vi "FindBlob_Pass1.vi"(0 "Image in":u32[][](graph), 1 "Connectivity":enum16{"4", "8"}(ring)) -> (2 "Image out":u32[][](graph), 3 "output array":u32[](array[numeric]), 4 "duplicates":cluster{u8, u8, u8}[](array[cluster]))   [LabVIEW 2024]
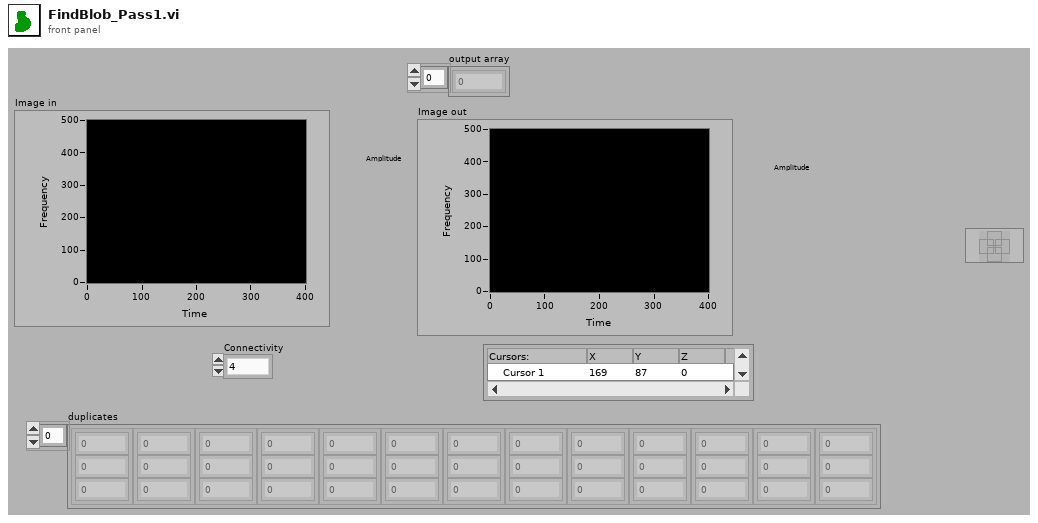
[diagram p1: front panel]
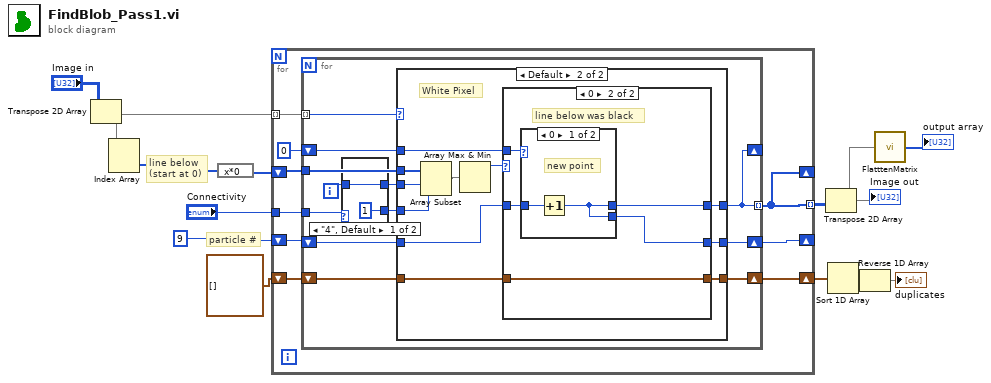
[diagram p0: block diagram]
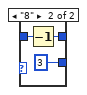
[diagram p2: hidden frame]
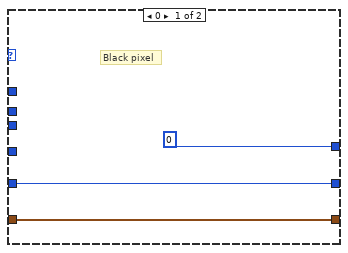
[diagram p3: hidden frame]
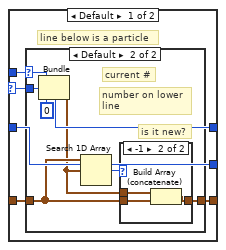
[diagram p4: hidden frame]
diagram:
  # "particle #"
  # "line below\n(start at 0)"
  n1 = Transpose 2D Array(2D array="Image in") -> (transposed array=w8:u32[][])
  n2 = Index Array(array=w8) -> (element=w9:u32[])  [unwired: 2 in]
  n3 = expression code="x*0"(w9) -> (w10:u32[])
  n4 = for {
    tunnel: w8 -> [w20] mode=indexing
    shift-right: [w21] -> _
    shift-left: u32 9 -> [w22]
    tunnel: [w18] -> w6 mode=indexing
    shift-right: [w18] -> _
    shift-left: w10 -> [w19]
    tunnel: "Connectivity" -> [w17]
    shift-right: [w15] -> w13
    shift-left: cluster{u8, u8, u8}[] [] -> [w16]
    n5 = for {
      tunnel: w20 -> [w34] mode=indexing
      shift-right: [w23] -> _
      shift-left: u32 0 -> [w33]
      shift-right: [w32] -> w21
      shift-left: w22 -> [w31]
      tunnel: [w23] -> w18 mode=indexing
      tunnel: w19 -> [w30]
      tunnel: w17 -> [w26]
      shift-right: [w24] -> w15
      shift-left: w16 -> [w25]
      i -> [w29]
      n6 = case shown="\"4\", Default" w26 {
        tunnel: w29 -> [w36 w39]
        tunnel: [w36 w38] -> w28
        tunnel: [1 ("length") 3 ("length")] -> w27
        frame "4", Default {
        }
        frame "8" {
          n7 = Decrement(x=w39) -> (x-1=w38:i32)
        }
      }
      n8 = case shown="Default" w34 {
        tunnel: w33 -> [_ w53]
        tunnel: [u8 0 w52] -> w23
        tunnel: [w42 w47] -> w32
        tunnel: w31 -> [w42 w46]
        tunnel: w30 -> [_ w51]
        tunnel: w28 -> [_ w50]
        tunnel: w27 -> [_ w45]
        tunnel: w25 -> [w40 w44]
        tunnel: [w40 w43] -> w24
        frame 0 {
          # "Black pixel"
        }
        frame Default {
          # "White Pixel"
          n9 = Array Subset(array=w51, index=w50, length=w45) -> (w49:u32[])
          n10 = Array Max & Min(array=w49) -> (max value=w48:u32)  [unwired: 3 out]
          n11 = case shown="0" w48 {
            selector: w48 -> [w58 _]
            tunnel: w53 -> [w54 w75]
            tunnel: w46 -> [w57 w74]
            tunnel: [w58 w73] -> w52
            tunnel: [w57 w71] -> w47
            tunnel: w44 -> [w55 w72]
            tunnel: [w56 w72] -> w43
            frame Default {
              # "line below is a particle"
              n12 = case shown="Default" w54 {
                selector: w54 -> [_ w61]
                tunnel: w58 -> [_ w66]
                tunnel: [w59 w65] -> w56
                tunnel: w55 -> [w59 w64]
                frame 0 {
                  # "beginning of a line"
                }
                frame Default {
                  # "is it new?"
                  # "number on lower\nline"
                  # "current #"
                  n13 = Bundle(w61, w66, u32 0) -> (w63:cluster{u32, u32, u32})  [unwired: 1 out]
                  n14 = Search 1D Array(1D array=w64, element=w63) -> (index of element=w62:i32)  [unwired: 1 out]
                  n15 = case shown="-1" w62 {
                    tunnel: [w67 w70] -> w65
                    tunnel: w64 -> [w67 w69]
                    tunnel: w63 -> [_ w68]
                    frame Default {
                    }
                    frame -1 {
                      n16 = Build Array (concatenate)(w68, w69) -> (w70:cluster{u32, u32, u32}[])
                    }
                  }
                }
              }
            }
            frame 0 {
              # "line below was black"
              n17 = case shown="0" w75 {
                selector: w75 -> [_ w79]
                tunnel: [w76 w79] -> w73
                tunnel: w74 -> [w77 w78]
                tunnel: [w76 w78] -> w71
                frame 0 {
                  # "new point"
                  n18 = Increment(x=w77) -> (x+1=w76:u32)
                }
                frame Default {
                  # "in a particle"
                }
              }
            }
          }
        }
      }
    }
  }
  n19 = Transpose 2D Array(2D array=w6) -> (transposed array=w4:u32[][])
  "Image out" <- w4
  n20 = Sort 1D Array(array=w13) -> (sorted array=w2:cluster{u32, u32, u32}[])
  n21 = Reverse 1D Array(array=w2) -> (reversed array=→"duplicates":cluster{u32, u32, u32}[])
  n22 = call <userlib>:"FlatttenMatrix.vi"("Matrix"=w4) -> ("Array"=→"output array":i32[])
